vi "Begin.vi"(1 "error in (no error)":errorcluster) -> (0 "error out":errorcluster)   [LabVIEW 2017]
doc: "Called before other user functions, this VI is expected to open initial I/O refnums, load in file data, and do all program initialization. Notice that the <B>error out</B> terminal is simply used for data flow. Wiring it to other structures or subVIs ensures that this VI runs first."
uses:
  <vilib>/Rock Robotics/WPI/Joystick/WPI_JoystickDeviceEnum.ctl
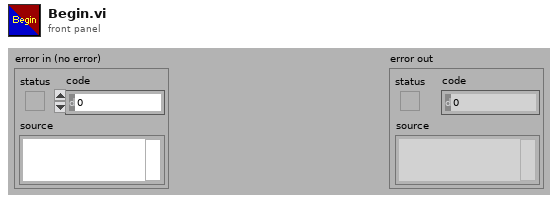
[diagram p1: front panel]
types:
  T1 = enum16{"swerve1", "swerve2", "swerve3", "swerve4"}[]
  T2 = typedef "WPI_JoystickDeviceEnum.ctl" = enum16{"USB 0", "USB 1", "USB 2", "USB 3", "USB 4", "USB 5"}
  T3 = typedef "WPI_MotorControlDeviceRef.ctl" = cluster{"DeviceStatus":errorcluster, "Type":T4, "PWM":cluster{"PWM Channel":T5, "DeadBand":T6}, "CAN":cluster{"Device Number":u8, "SetOutput VI Ref":variant, "GetOutput VI Ref":variant, "Enable VI Ref":variant, "Disable VI Ref":variant, "Data":variant}, "Invert":bool, "DIO PWM":cluster{"PWM \"Enable\" Channel":T5, "DIOChannel":T7, "PWM Rate":dbl}}
  T4 = typedef "WPI_MotorControlType.ctl" = enum16{"PWM", "CAN", "DIO PWM"}
  T5 = typedef "FPGA_DIOPWMChannel.ctl" = enum8{"PWM 0", "PWM 1", "PWM 2", "PWM 3", "PWM 4", "PWM 5", "PWM 6", "PWM 7", "PWM 8", "PWM 9", "PWM MXP 0", "PWM MXP 1", "PWM MXP 2", "PWM MXP 3", "PWM MXP 4", "PWM MXP 5", "PWM MXP 6", "PWM MXP 7", "PWM MXP 8", "PWM MXP 9", "Invalid"}
  T6 = typedef "WPI_PWMDeadband.ctl" = cluster{"Name":string, "maxPositivePwm":i32, "minPositivePwm":i32, "centerPwm":i32, "maxNegativePwm":i32, "minNegativePwm":i32, "angularRange":u16}
  T7 = typedef "FPGA_DIOChannel.ctl" = enum8{"DIO 0", "DIO 1", "DIO 2", "DIO 3", "DIO 4", "DIO 5", "DIO 6", "DIO 7", "DIO 8", "DIO 9", "DIO MXP 0", "DIO MXP 1", "DIO MXP 2", "DIO MXP 3", "DIO MXP 4", "DIO MXP 5", "DIO MXP 6", "DIO MXP 7", "DIO MXP 8", "DIO MXP 9", "DIO MXP 10", "DIO MXP 11", "DIO MXP 12", "DIO MXP 13", "DIO MXP 14", "DIO MXP 15", "SPI Port CS1", "SPI Port CS2", "SPI Port CS3", "SPI Port MISO", "SPI Port MOSI", "Invalid"}
  T8 = typedef "WPI_JoystickDevRef.ctl" = cluster{"Device":T2}
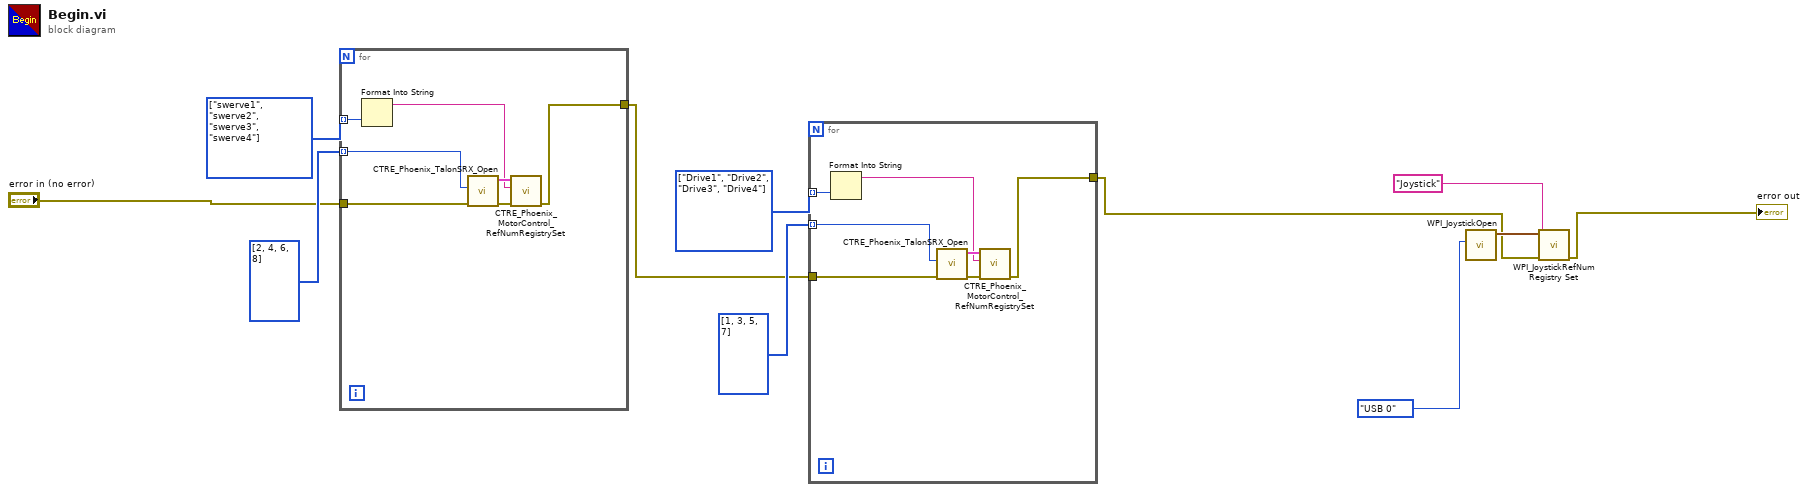
[diagram p0: block diagram]
diagram:
  w6 = enum16{"Drive1", "Drive2", "Drive3", "Drive4"}[] [enum."Drive1", enum."Drive2", enum."Drive3", enum."Drive4"] items=["Drive1", "Drive2", "Drive3", "Drive4"]
  w9 = T1 [enum."swerve1", enum."swerve2", enum."swerve3", enum."swerve4"] items=["swerve1", "swerve2", "swerve3", "swerve4"]
  n1 = for {
    tunnel: w9 -> [w16] mode=indexing
    tunnel: u8[] [2, 4, 6, 8] -> [w14] mode=indexing
    tunnel: "error in (no error)" -> [w13]
    tunnel: [w12] -> w4
    n2 = Format Into String(w16) -> (resulting string=w15:string)  [unwired: 3 in, 1 out]
    n3 = call <vilib>:"CTRE_Phoenix_TalonSRX_Open.vi"("error in"=w13, "Device Number"=w14) -> ("error out"=w17:errorcluster, "CAN Talon SRX Ref"=w18:T3)  [unwired: 8 in]
    n4 = call <vilib>:"CTRE_Phoenix_MotorControl_RefNumRegistrySet.vi"("error in (no error)"=w17, "refnum name"=w15, "PhoenixMotorControlDevRef"=w18) -> ("error out"=w12:errorcluster)  [unwired: 7 in, 1 out]
  }
  n5 = for {
    tunnel: w6 -> [w23] mode=indexing
    tunnel: u8[] [1, 3, 5, 7] -> [w21] mode=indexing
    tunnel: w4 -> [w20]
    tunnel: [w19] -> w3
    n6 = Format Into String(w23) -> (resulting string=w22:string)  [unwired: 3 in, 1 out]
    n7 = call <vilib>:"CTRE_Phoenix_TalonSRX_Open.vi"("error in"=w20, "Device Number"=w21) -> ("error out"=w24:errorcluster, "CAN Talon SRX Ref"=w25:T3)  [unwired: 8 in]
    n8 = call <vilib>:"CTRE_Phoenix_MotorControl_RefNumRegistrySet.vi"("error in (no error)"=w24, "refnum name"=w22, "PhoenixMotorControlDevRef"=w25) -> ("error out"=w19:errorcluster)  [unwired: 7 in, 1 out]
  }
  n9 = call <vilib>:"WPI_JoystickOpen.vi"("JoystickDevice"=WPI_JoystickDeviceEnum."USB 0") -> ("JoystickDevRef"=w11:T8)  [unwired: 10 in]
  n10 = call <vilib>:"WPI_JoystickRefNum Registry Set.vi"("error in (no error)"=w3, "refnum name"="Joystick", "JoystickDevRef"=w11) -> ("error out"=→"error out":errorcluster)  [unwired: 7 in, 1 out]
